vi "例7-3(2).vi"() -> ()   [LabVIEW 2019]
panel:
  in  "IP":string="LocalHost"
  in  "端口":u16=6040
  in  "停止按钮":bool
  out "波形图（客户机）":dbl[](graph)
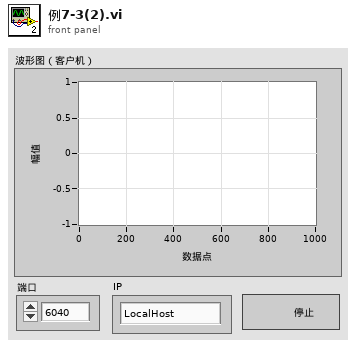
[diagram p1: front panel]
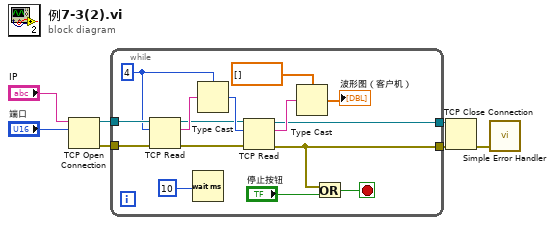
[diagram p0: block diagram]
diagram:
  n1 = TCP Open Connection(address="IP", remote port or service name="端口") -> (connection ID=w6:refnum<k5>, error out=w5:errorcluster)  [unwired: 3 in]
  n2 = while {
    tunnel: w6 -> [w22]
    tunnel: w5 -> [w21]
    tunnel: [w12] -> w4
    tunnel: [w11] -> w3
    stop <- w9 stop-if-true
    w18 = 4
    n3 = TCP Read(connection ID=w22, bytes to read=w18, error in (no error)=w21) -> (connection ID out=w17:refnum<k5>, data out=w20:string, error out=w16:errorcluster)  [unwired: 2 in]
    n4 = Wait (ms)(milliseconds to wait=10) -> ()  [unwired: 1 out]
    n5 = Type Cast(type=w18, x=w20) -> (*(type *) &x=w19:i32)
    n6 = TCP Read(connection ID=w17, bytes to read=w19, error in (no error)=w16) -> (connection ID out=w12:refnum<k5>, data out=w14:string, error out=w11:errorcluster)  [unwired: 2 in]
    n7 = Type Cast(type=dbl[] [], x=w14) -> (*(type *) &x=→"波形图（客户机）":dbl[])
    n8 = Or(x=w11, y="停止按钮") -> (x .or. y?=w9:bool)
  }
  n9 = TCP Close Connection(connection ID=w4, error in (no error)=w3) -> (error out=w2:errorcluster)  [unwired: 1 in, 1 out]
  n10 = call <vilib>:"Simple Error Handler.vi"("error in (no error)"=w2) -> ()  [unwired: 4 in, 5 out]
